vi "Write Parent Attributes.vi"(10 "Parent Attributes":refnum<data-value>, 11 "TEMPLATE Actor in":refnum<class "TEMPLATE Actor.lvclass">) -> (3 "TEMPLATE Actor out":refnum<class "TEMPLATE Actor.lvclass">)   [LabVIEW 2020, in "_Template.lvlib" / "Templates.lvlib" / "TEMPLATE jettl Actor.lvlib" / "TEMPLATE Actor.lvlib" / "TEMPLATE Actor.lvclass"]
uses:
  TEMPLATE Actor.lvclass
  TEMPLATE Actor.lvclass/TEMPLATE Actor.ctl
  jettl/jettl/Actor/Actor.lvclass
  jettl/jettl/Transport/Transport.lvclass
  jettl/jettl/Msg/Msg.lvclass
  jettl/jettl/Msgs.ctl
  jettl/jettl/jettl.lvlib
  jettl/jettl/Attributes Metadata/Attributes Metadata.lvclass
  jettl/jettl/Attributes.ctl
panel:
  # "This front panel should not be manipulated."
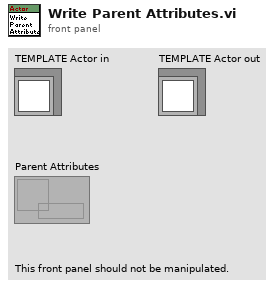
[diagram p1: front panel]
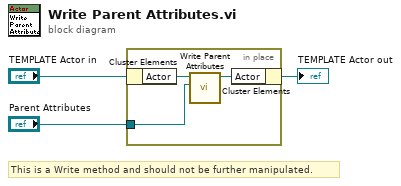
[diagram p0: block diagram]
diagram:
  # "This is a Write method and should not be further manipulated."
  n1 = in-place {
    in-place-border: "Parent Attributes" -> [w4]
    n2 = in-place-cluster #1("TEMPLATE Actor in") -> ("Actor"=w6:refnum<class "Actor.lvclass">)
    n3 = call-dynamic "Write Parent Attributes.vi"("Parent Attributes"=w4, "Actor in"=w6) -> ("Actor out"=w5:refnum<class "Actor.lvclass">)  [unwired: 9 in]
    n4 = in-place-cluster #1("Actor"=w5) -> (→"TEMPLATE Actor out":refnum<class "TEMPLATE Actor.lvclass">)
  }
